vi "Agilent PWM Set Blank Screen.vi"(7 "Agilent PWM":T1, 8 "error in (no error)":errorcluster, 10 "Blank Screen":bool, 11 "VISA Resource Name":refnum<visa-resource-name>) -> (0 "error out":errorcluster, 3 "dup VISA Resource Name":refnum<visa-resource-name>)   [LabVIEW 2011]
doc: "This VI for the HP 8753 is used to read the sweep type.\n\n0 LINEAR FREQ\n1 LOG FREQ\n2 LIST FREQ\n3 CW TIME\n4 POWER SWEEP"
uses:
  TypeDefs/Agilent PWM Instrument Info.ctl
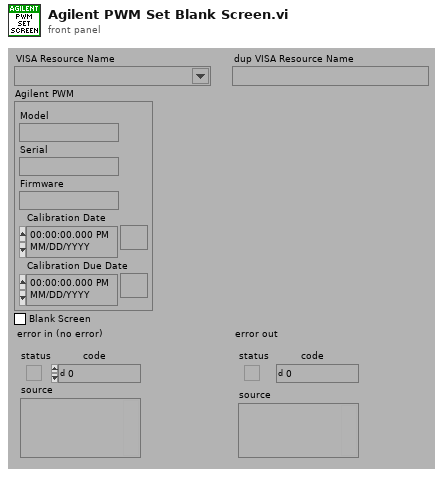
[diagram p1: front panel]
types:
  T1 = typedef "Agilent PWM Instrument Info.ctl" = cluster{"Model":string, "Serial":string, "Firmware":string, "Calibration Date":timestamp, "Calibration Due Date":timestamp}
  T2 = typedef "Agilent PWM Model.ctl" = enum16{"Not Supported", "E4418X", "E4419X", "U2000X"}
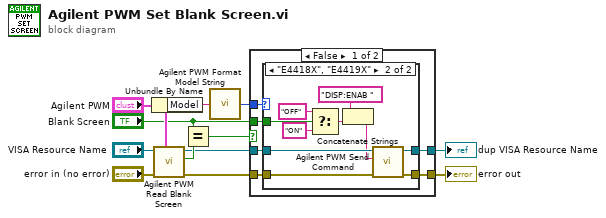
[diagram p0: block diagram]
diagram:
  n1 = Unbundle By Name("Agilent PWM") -> ("Model"=w9:string)
  n2 = call "Agilent PWM Read Blank Screen.vi"("Agilent PWM"="Agilent PWM", "error in (no error)"="error in (no error)", "VISA Resource Name"="VISA Resource Name") -> ("error out"=w5:errorcluster, "Blank Screen"=w10:bool, "dup VISA Resource Name"=w6:refnum<visa-resource-name>)  [unwired: 6 out]
  n3 = Equal?(x="Blank Screen", y=w10) -> (x = y?=w1:bool)
  n4 = call "Agilent PWM Format Model String.vi"("Model"=w9) -> ("Model"=w2:T2)
  n5 = case shown="False" w1 {
    tunnel: [w18 w32] -> w4
    tunnel: [w17 w31] -> w3
    tunnel: w6 -> [w16 w32]
    tunnel: w5 -> [w15 w31]
    tunnel: "Blank Screen" -> [w14 _]
    tunnel: w2 -> [w13 _]
    frame False {
      n6 = case shown="\"E4418X\", \"E4419X\"" w13 {
        tunnel: [w20 w30] -> w18
        tunnel: [w19 w29] -> w17
        tunnel: w16 -> [w20 w28]
        tunnel: w15 -> [w19 w27]
        tunnel: w14 -> [_ w21]
        frame "Not Supported", "U2000X" {
        }
        frame "E4418X", "E4419X" {
          n7 = Select(t="OFF" ("write buffer"), s=w21, f="ON" ("write buffer")) -> (s? t:f=w26:string)
          n8 = Concatenate Strings("DISP:ENAB " ("string"), w26) -> (w22:string)
          n9 = call "Agilent PWM Send Command.vi"("error in (no error)"=w27, "Command"=w22, "VISA Resource Name"=w28) -> ("error out"=w29:errorcluster, "dup VISA Resource Name"=w30:refnum<visa-resource-name>)  [unwired: 2 in, 5 out]
        }
      }
    }
    frame True {
    }
  }
  "dup VISA Resource Name" <- w4
  "error out" <- w3
